vi "Parse Sentence_RMC.vi"(8 "error in (no error)":errorcluster, 11 "RMC sentence":string) -> (0 "error out":errorcluster, 3 "RMC_Data":T1 {"status"."value" items=["Void", "Active"]; "type of fix"."mode" items=["Simulator", "Not Valid", "Estimated", "Differential", "Autonomous"]})   [LabVIEW 2024]
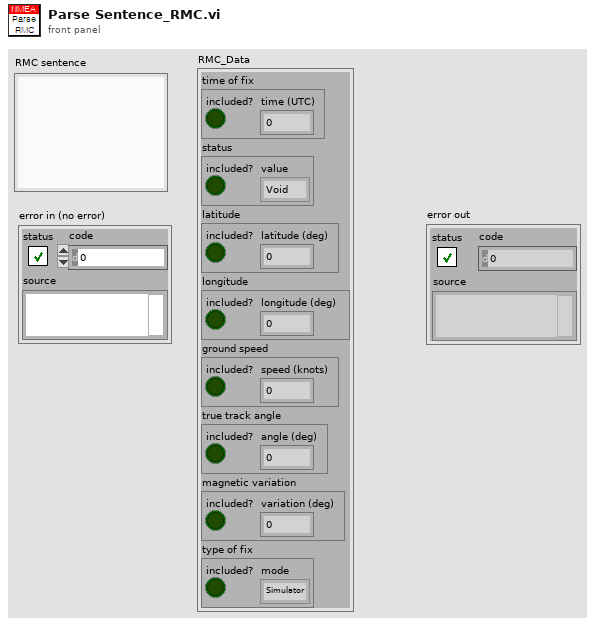
[diagram p1: front panel]
types:
  T1 = cluster{"time of fix":cluster{"included?":bool, "time (UTC)":dbl}, "status":cluster{"included?":bool, "value":u16}, "latitude":cluster{"included?":bool, "latitude (deg)":dbl}, "longitude":cluster{"included?":bool, "longitude (deg)":dbl}, "ground speed":cluster{"included?":bool, "speed (knots)":dbl}, "true track angle":cluster{"included?":bool, "angle (deg)":dbl}, "magnetic variation":cluster{"included?":bool, "variation (deg)":dbl}, "type of fix":cluster{"included?":bool, "mode":u16}}
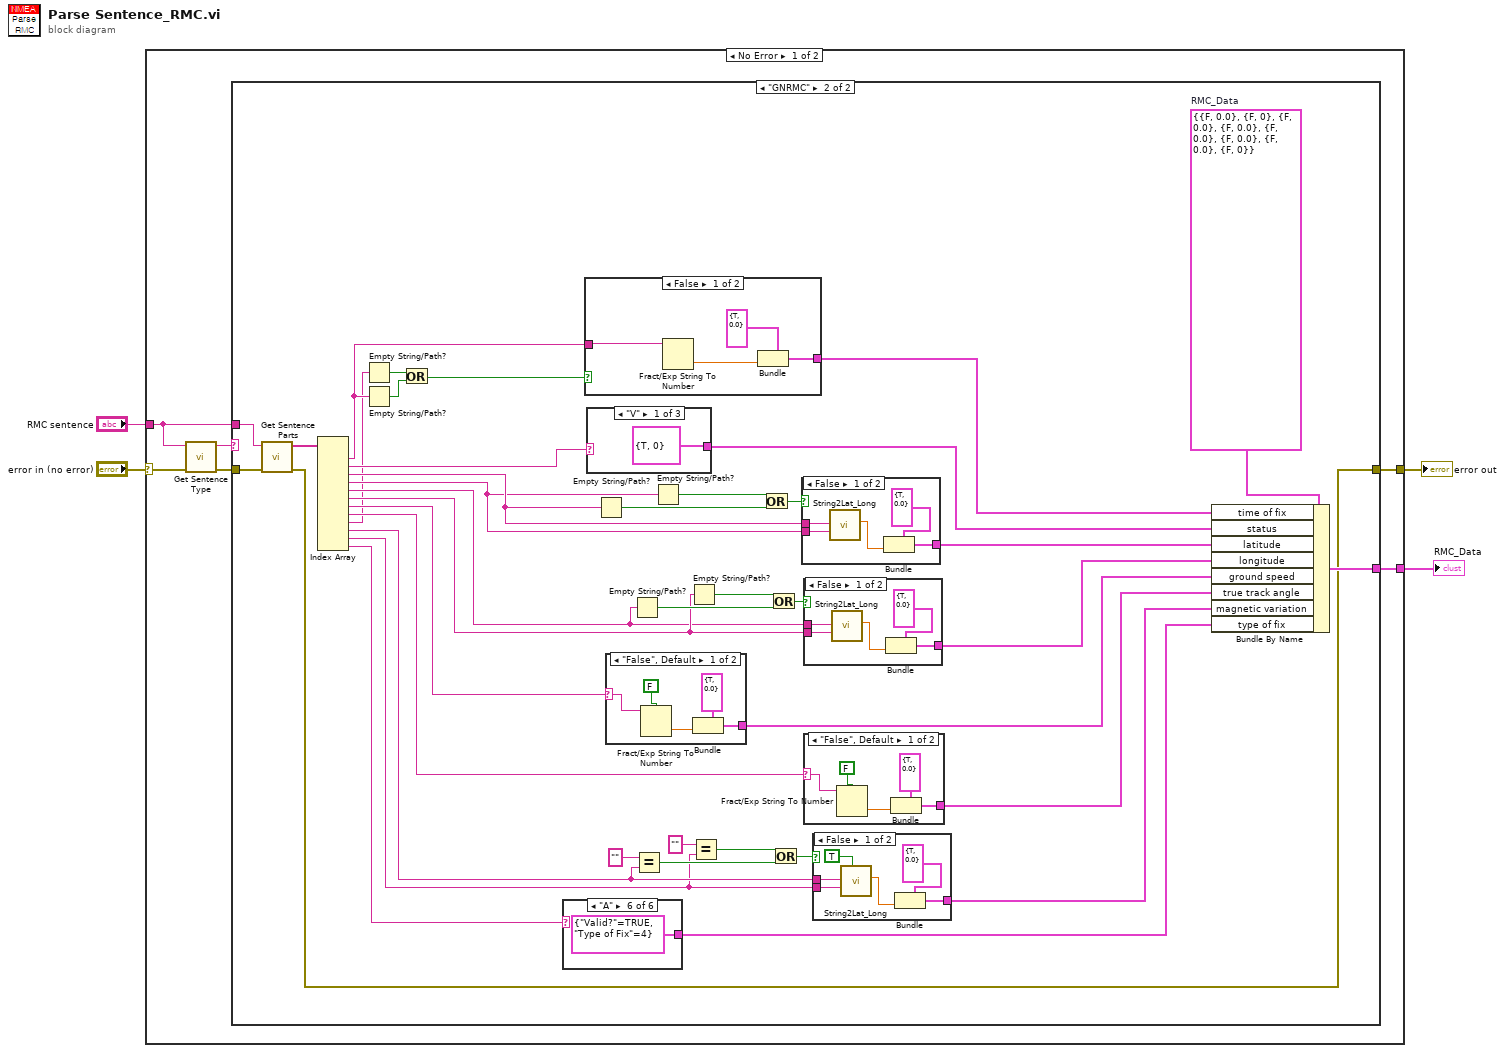
[diagram p0: block diagram]
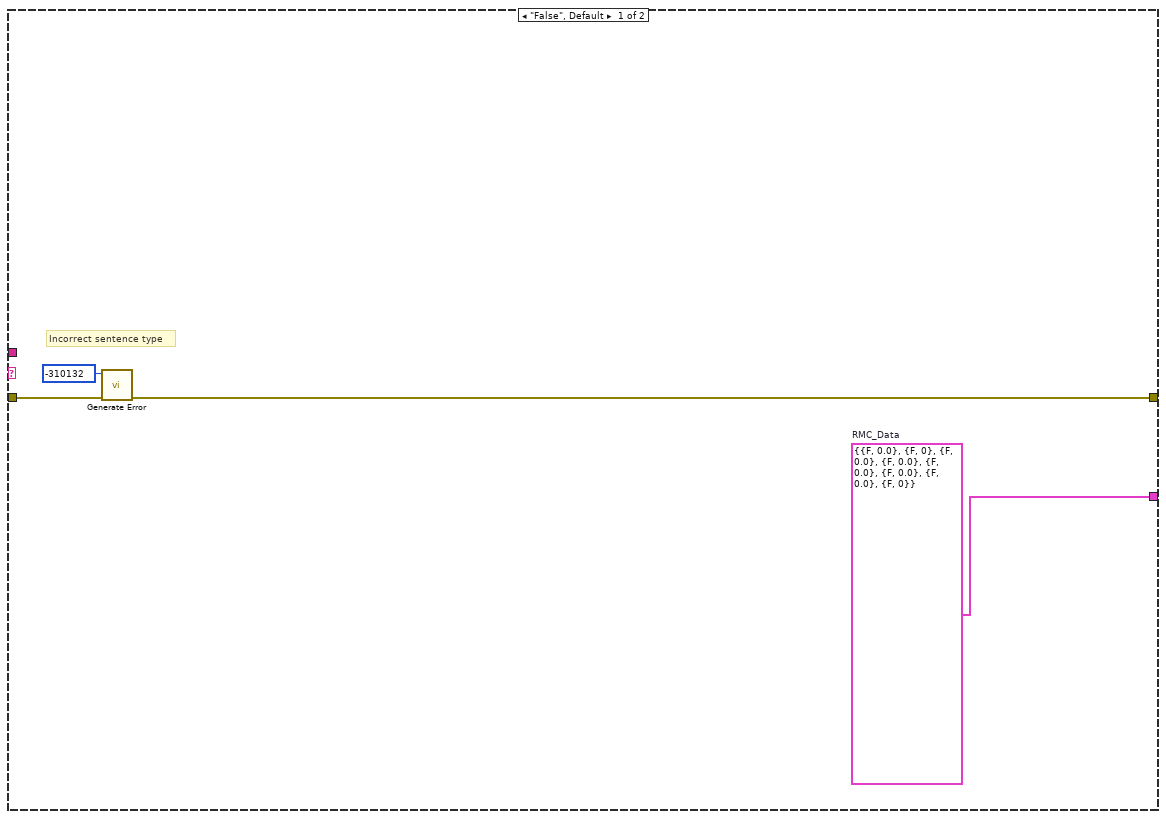
[diagram p2: hidden frame]
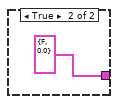
[diagram p3: hidden frame]
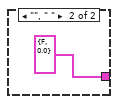
[diagram p4: hidden frame]
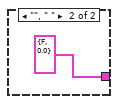
[diagram p5: hidden frame]
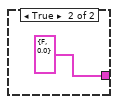
[diagram p6: hidden frame]
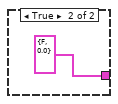
[diagram p7: hidden frame]
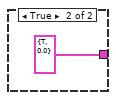
[diagram p8: hidden frame]
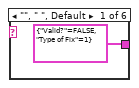
[diagram p9: hidden frame]
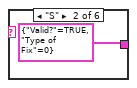
[diagram p10: hidden frame]
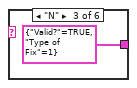
[diagram p11: hidden frame]
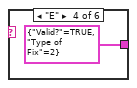
[diagram p12: hidden frame]
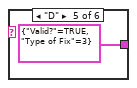
[diagram p13: hidden frame]
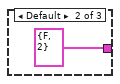
[diagram p14: hidden frame]
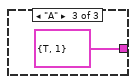
[diagram p15: hidden frame]
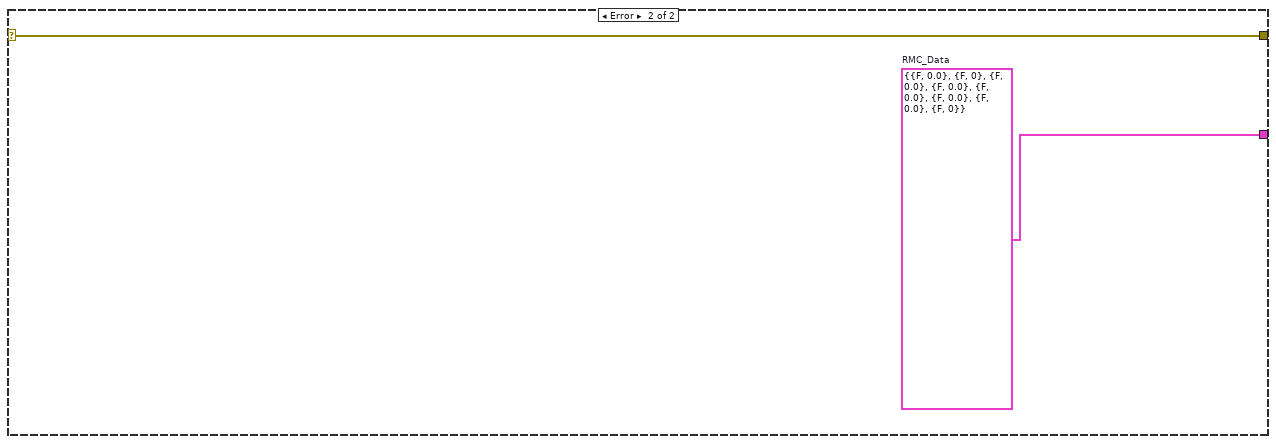
[diagram p16: hidden frame]
diagram:
  n1 = case shown="No Error" "error in (no error)" {
    selector: "error in (no error)" -> [w8 w101]
    tunnel: [w9 w101] -> w2
    tunnel: [w10 w100] -> w1
    tunnel: "RMC sentence" -> [w6 _]
    frame No Error {
      n2 = call "Get Sentence Type.vi"("error in (no error)"=w8, "sentence"=w6) -> ("error out"=w7:errorcluster, "sentence type"=w5:string)  [unwired: 7 in, 1 out]
      n3 = case shown="\"GNRMC\"" w5 {
        tunnel: w6 -> [_ w20]
        tunnel: w7 -> [w13 w54]
        tunnel: [w11 w53] -> w10
        tunnel: [w12 w18] -> w9
        frame "False", Default {
          w11 = T1 {"time of fix"={"included?"=FALSE, "time (UTC)"=0.0}, "status"={"included?"=FALSE, "value"=0}, "latitude"={"included?"=FALSE, "latitude (deg)"=0.0}, "longitude"={"included?"=FALSE, "longitude (deg)"=0.0}, "ground speed"={"included?"=FALSE, "speed (knots)"=0.0}, "true track angle"={"included?"=FALSE, "angle (deg)"=0.0}, "magnetic variation"={"included?"=FALSE, "variation (deg)"=0.0}, "type of fix"={"included?"=FALSE, "mode"=0}}  # RMC_Data
          # "Incorrect sentence type"
          n4 = call "Generate Error.vi"("error in (no error)"=w13, "code"=-310132) -> ("error out"=w12:errorcluster)  [unwired: 9 in]
        }
        frame "GNRMC" {
          w15 = T1 {"time of fix"={"included?"=FALSE, "time (UTC)"=0.0}, "status"={"included?"=FALSE, "value"=0}, "latitude"={"included?"=FALSE, "latitude (deg)"=0.0}, "longitude"={"included?"=FALSE, "longitude (deg)"=0.0}, "ground speed"={"included?"=FALSE, "speed (knots)"=0.0}, "true track angle"={"included?"=FALSE, "angle (deg)"=0.0}, "magnetic variation"={"included?"=FALSE, "variation (deg)"=0.0}, "type of fix"={"included?"=FALSE, "mode"=0}}  # RMC_Data
          n5 = call "Get Sentence Parts.vi"("error in (no error)"=w54, "sentence"=w20) -> ("error out"=w18:errorcluster, "sentence data"=w19:string[])  [unwired: 7 in, 1 out]
          n6 = Index Array(array=w19) -> (element #1=w47:string, element #2=w52:string, element #3=w43:string, element #4=w42:string, element #5=w33:string, element #6=w34:string, element #7=w32:string, element #8=w30:string, element #9=w17:string, element #10=w23:string, element #11=w22:string, element #12=w51:string)  [unwired: 12 in]
          n7 = Empty String/Path?(string/path=w17) -> (empty?=w49:bool)
          n8 = Empty String/Path?(string/path=w47) -> (empty?=w50:bool)
          n9 = Or(x=w49, y=w50) -> (x .or. y?=w48:bool)
          n10 = case shown="\"A\"" w51 {
            tunnel: [cluster{"Valid?":bool, "Type of Fix":u16} {"Valid?"=FALSE, "Type of Fix"=1} ("Type of Fix") cluster{"Valid?":bool, "Type of Fix":u16} {"Valid?"=TRUE, "Type of Fix"=0} ("Type of Fix") cluster{"Valid?":bool, "Type of Fix":u16} {"Valid?"=TRUE, "Type of Fix"=1} ("Type of Fix") cluster{"Valid?":bool, "Type of Fix":u16} {"Valid?"=TRUE, "Type of Fix"=2} ("Type of Fix") cluster{"Valid?":bool, "Type of Fix":u16} {"Valid?"=TRUE, "Type of Fix"=3} ("Type of Fix") cluster{"Valid?":bool, "Type of Fix":u16} {"Valid?"=TRUE, "Type of Fix"=4} ("Type of Fix")] -> w21
            frame "", " ", Default {
            }
            frame "S" {
            }
            frame "N" {
            }
            frame "E" {
            }
            frame "D" {
            }
            frame "A" {
            }
          }
          n11 = case shown="False" w48 {
            tunnel: [w89 cluster{"Valid?":bool, "Latitude (Deg)":dbl} {"Valid?"=TRUE, "Latitude (Deg)"=0.0} ("time of fix")] -> w46
            tunnel: w47 -> [w88 _]
            frame False {
              n12 = Fract/Exp String To Number(string=w88) -> (number=w87:dbl)  [unwired: 4 out]
              n13 = Bundle(cluster=cluster{"Valid?":bool, "Latitude (Deg)":dbl} {"Valid?"=TRUE, "Latitude (Deg)"=0.0} ("time of fix"), "Latitude (Deg)"=w87) -> (w89:cluster{"Valid?":bool, "Latitude (Deg)":dbl})  [unwired: 1 out]
            }
            frame True {
            }
          }
          n14 = case shown="\"V\"" w52 {
            tunnel: [cluster{"Valid?":bool, "Status":u16} {"Valid?"=TRUE, "Status"=0} ("Status") cluster{"Valid?":bool, "Status":u16} {"Valid?"=FALSE, "Status"=2} ("Status") cluster{"Valid?":bool, "Status":u16} {"Valid?"=TRUE, "Status"=1} ("Status")] -> w41
            frame "V" {
            }
            frame Default {
            }
            frame "A" {
            }
          }
          n15 = Empty String/Path?(string/path=w43) -> (empty?=w44:bool)
          n16 = case shown="\"False\", Default" w32 {
            selector: w32 -> [w72 _]
            tunnel: [w69 cluster{"Valid?":bool, "Speed (Knots)":dbl} {"Valid?"=FALSE, "Speed (Knots)"=0.0} ("Ground Speed")] -> w31
            frame "False", Default {
              n17 = Fract/Exp String To Number(use system decimal point (T)=FALSE, string=w72) -> (number=w70:dbl)  [unwired: 3 out]
              n18 = Bundle(cluster=cluster{"Valid?":bool, "Speed (Knots)":dbl} {"Valid?"=TRUE, "Speed (Knots)"=0.0} ("Ground Speed"), "Speed (Knots)"=w70) -> (w69:cluster{"Valid?":bool, "Speed (Knots)":dbl})  [unwired: 1 out]
            }
            frame "", " " {
            }
          }
          n19 = Empty String/Path?(string/path=w33) -> (empty?=w37:bool)
          n20 = Equal?(x="", y=w23) -> (x = y?=w25:bool)
          n21 = Empty String/Path?(string/path=w42) -> (empty?=w45:bool)
          n22 = Empty String/Path?(string/path=w34) -> (empty?=w36:bool)
          n23 = Equal?(x="", y=w22) -> (x = y?=w26:bool)
          n24 = Or(x=w45, y=w44) -> (x .or. y?=w40:bool)
          n25 = Or(x=w36, y=w37) -> (x .or. y?=w35:bool)
          n26 = Or(x=w26, y=w25) -> (x .or. y?=w24:bool)
          n27 = case shown="False" w40 {
            tunnel: w43 -> [w84 _]
            tunnel: w42 -> [w83 _]
            tunnel: [w80 cluster{"Valid?":bool, "Latitude (Deg)":dbl} {"Valid?"=FALSE, "Latitude (Deg)"=0.0} ("Latitude")] -> w39
            frame False {
              n28 = call "String2Lat_Long.vi"("direction string"=w83, "numeric string for lat/lon"=w84) -> ("composite value"=w82:dbl)  [unwired: 9 in]
              n29 = Bundle(cluster=cluster{"Valid?":bool, "Latitude (Deg)":dbl} {"Valid?"=TRUE, "Latitude (Deg)"=0.0} ("Latitude"), "Latitude (Deg)"=w82) -> (w80:cluster{"Valid?":bool, "Latitude (Deg)":dbl})  [unwired: 1 out]
            }
            frame True {
            }
          }
          n30 = case shown="False" w35 {
            tunnel: w33 -> [w78 _]
            tunnel: w34 -> [w77 _]
            tunnel: [w74 cluster{"Valid?":bool, "Latitude (Deg)":dbl} {"Valid?"=FALSE, "Latitude (Deg)"=0.0} ("Latitude")] -> w38
            frame False {
              n31 = call "String2Lat_Long.vi"("direction string"=w77, "numeric string for lat/lon"=w78) -> ("composite value"=w76:dbl)  [unwired: 9 in]
              n32 = Bundle(cluster=cluster{"Valid?":bool, "Latitude (Deg)":dbl} {"Valid?"=TRUE, "Latitude (Deg)"=0.0} ("Latitude"), "Latitude (Deg)"=w76) -> (w74:cluster{"Valid?":bool, "Latitude (Deg)":dbl})  [unwired: 1 out]
            }
            frame True {
            }
          }
          n33 = case shown="\"False\", Default" w30 {
            selector: w30 -> [w66 _]
            tunnel: [w63 cluster{"Valid?":bool, "Speed (Knots)":dbl} {"Valid?"=FALSE, "Speed (Knots)"=0.0} ("Ground Speed")] -> w29
            frame "False", Default {
              n34 = Fract/Exp String To Number(use system decimal point (T)=FALSE, string=w66) -> (number=w64:dbl)  [unwired: 3 out]
              n35 = Bundle(cluster=cluster{"Valid?":bool, "Speed (Knots)":dbl} {"Valid?"=TRUE, "Speed (Knots)"=0.0} ("Ground Speed"), "Speed (Knots)"=w64) -> (w63:cluster{"Valid?":bool, "Speed (Knots)":dbl})  [unwired: 1 out]
            }
            frame "", " " {
            }
          }
          n36 = case shown="False" w24 {
            tunnel: w23 -> [w60 _]
            tunnel: w22 -> [w59 _]
            tunnel: [w56 cluster{"Valid?":bool, "Latitude (Deg)":dbl} {"Valid?"=FALSE, "Latitude (Deg)"=0.0} ("Latitude")] -> w16
            frame False {
              n37 = call "String2Lat_Long.vi"("magnetic variation?"=TRUE ("Magnetic Variation?"), "direction string"=w59, "numeric string for lat/lon"=w60) -> ("composite value"=w58:dbl)  [unwired: 8 in]
              n38 = Bundle(cluster=cluster{"Valid?":bool, "Latitude (Deg)":dbl} {"Valid?"=TRUE, "Latitude (Deg)"=0.0} ("Latitude"), "Latitude (Deg)"=w58) -> (w56:cluster{"Valid?":bool, "Latitude (Deg)":dbl})  [unwired: 1 out]
            }
            frame True {
            }
          }
          n39 = Bundle By Name(cluster=w15, "time of fix"=w46, "status"=w41, "latitude"=w39, "longitude"=w38, "ground speed"=w31, "true track angle"=w29, "magnetic variation"=w16, "type of fix"=w21) -> (w53:T1)
        }
      }
    }
    frame Error {
      w100 = T1 {"time of fix"={"included?"=FALSE, "time (UTC)"=0.0}, "status"={"included?"=FALSE, "value"=0}, "latitude"={"included?"=FALSE, "latitude (deg)"=0.0}, "longitude"={"included?"=FALSE, "longitude (deg)"=0.0}, "ground speed"={"included?"=FALSE, "speed (knots)"=0.0}, "true track angle"={"included?"=FALSE, "angle (deg)"=0.0}, "magnetic variation"={"included?"=FALSE, "variation (deg)"=0.0}, "type of fix"={"included?"=FALSE, "mode"=0}}  # RMC_Data
    }
  }
  "error out" <- w2
  "RMC_Data" <- w1
